vi "Read Name.vi"(8 "error in (no error)":errorcluster, 11 "Payload in":refnum<class "Payload.lvclass">) -> (0 "error out":errorcluster, 2 "Name":string, 3 "Payload out":refnum<class "Payload.lvclass">)   [LabVIEW 2015, in "Payload.lvclass"]
uses:
  Payload.lvclass
  Payload.lvclass/Payload.ctl
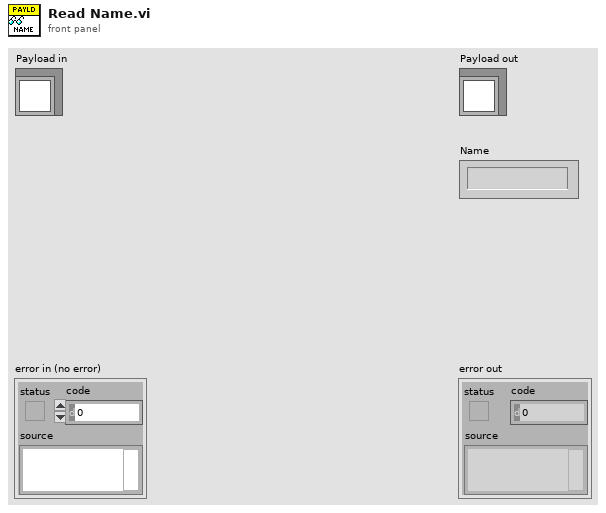
[diagram p1: front panel]
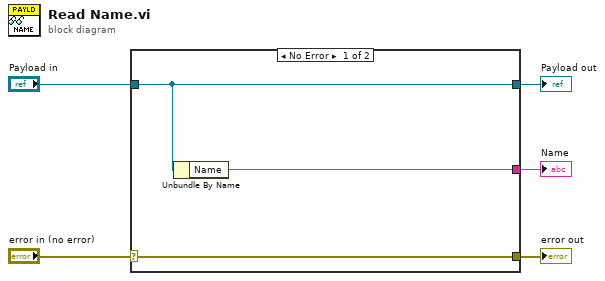
[diagram p0: block diagram]
diagram:
  n1 = case shown="No Error" "error in (no error)" {
    selector: "error in (no error)" -> [w8 w9]
    tunnel: [w8 w9] -> w4
    tunnel: [w7 w10] -> w2
    tunnel: "Payload in" -> [w7 w10]
    tunnel: [w6 _] -> w1
    frame No Error {
      n2 = Unbundle By Name(w7) -> ("Name"=w6:string)
    }
    frame Error {
    }
  }
  "error out" <- w4
  "Payload out" <- w2
  "Name" <- w1
